vi "combine two dist.vi"(6 "Array3":dbl[](array[numeric]), 9 "# bins":i32, 10 "Array2":dbl[](array[numeric]), 11 "Array1":dbl[](array[numeric])) -> (1 "Histogram 3":T1(graph), 2 "Histogram 2":T1(graph), 3 "Histogram 1":T1(graph))   [LabVIEW 2023]
uses:
  <vilib>/Analysis/NI_AALPro.lvlib
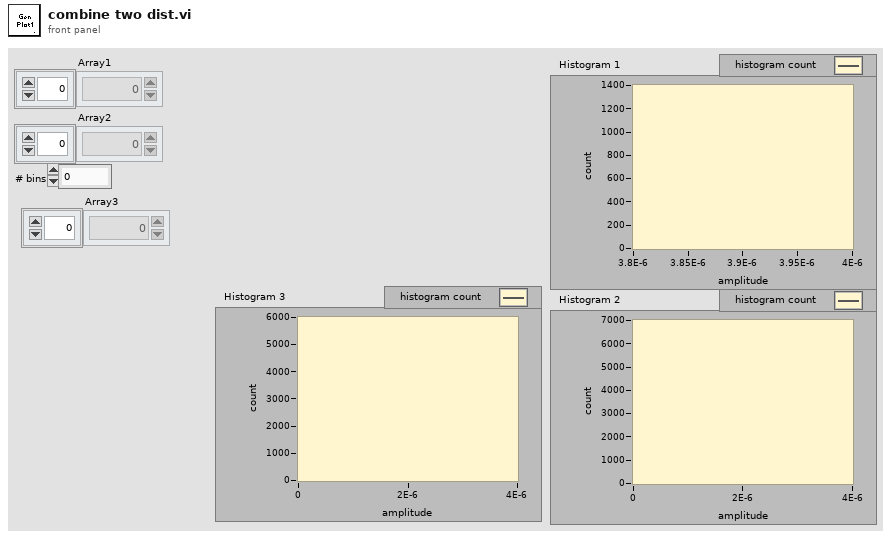
[diagram p1: front panel]
types:
  T1 = cluster{"X Values":dbl[], "Histogram: h(x)":i32[]}
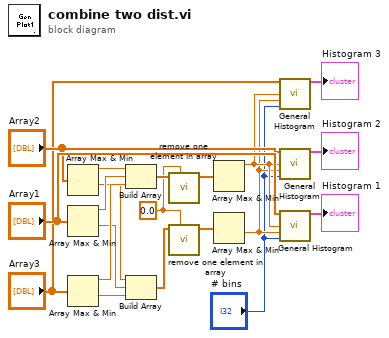
[diagram p0: block diagram]
diagram:
  w3 = 0.0 ("element to remove")
  n1 = Array Max & Min(array="Array2") -> (max value=w16:dbl, min value=w11:dbl)  [unwired: 2 out]
  n2 = Array Max & Min(array="Array1") -> (max value=w15:dbl, min value=w10:dbl)  [unwired: 2 out]
  n3 = Array Max & Min(array="Array3") -> (max value=w14:dbl, min value=w9:dbl)  [unwired: 2 out]
  n4 = Build Array(w16, w15, w14) -> (w5:dbl[])
  n5 = Build Array(w11, w10, w9) -> (w2:dbl[])
  n6 = call "remove one element in array.vi"("element to remove"=w3, "Input"=w5) -> ("Output"=w4:dbl[])  [unwired: 9 in]
  n7 = call "remove one element in array.vi"("element to remove"=w3, "Input"=w2) -> ("Output"=w1:dbl[])  [unwired: 9 in]
  n8 = Array Max & Min(array=w4) -> (max value=w12:dbl)  [unwired: 3 out]
  n9 = Array Max & Min(array=w1) -> (min value=w8:dbl)  [unwired: 3 out]
  n10 = call <vilib>:"General Histogram.vi"("X"="Array3", "max"=w12, "min"=w8, "# bins"="# bins") -> ("Histogram Graph"=→"Histogram 3":T1)  [unwired: 7 in, 4 out]
  n11 = call <vilib>:"General Histogram.vi"("X"="Array2", "max"=w12, "min"=w8, "# bins"="# bins") -> ("Histogram Graph"=→"Histogram 2":T1)  [unwired: 7 in, 4 out]
  n12 = call <vilib>:"General Histogram.vi"("X"="Array1", "max"=w12, "min"=w8, "# bins"="# bins") -> ("Histogram Graph"=→"Histogram 1":T1)  [unwired: 7 in, 4 out]
